vi "PXI-Update AO (Queue).vi"(0 "AO Tasks":T2[](array[typedef]), 5 "Wait for Buffer Space (T)?":bool=TRUE, 7 "AO Waveforms":dbl[][](array[numeric]), 11 "error in (no error)":errorcluster, 12 "DAQ Write State":T1) -> (14 "DAQ Write State Out":T1, 15 "error out":errorcluster)   [LabVIEW 2020]
uses:
  Type Defs/Task Struct.ctl
  Type Defs/DAQ Write State enum.ctl
  PXI Globals.vi
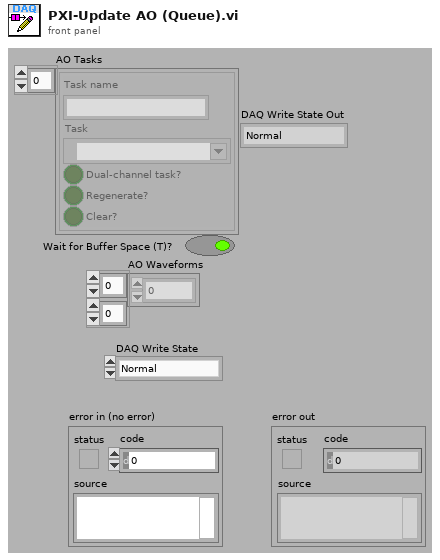
[diagram p1: front panel]
types:
  T1 = typedef "DAQ Write State enum.ctl" = enum16{"Normal", "Ramp down", "Zero buffers", "Done"}
  T2 = typedef "Task Struct.ctl" = cluster{"Task name":string, "Task":refnum<k21>, "Dual-channel task?":bool, "Regenerate?":bool, "Clear?":bool}
  T3 = typedef "Ramping Params.ctl" = cluster{"Ramp up?":bool, "Ramp down?":bool, "Ramp duration (msecs)":dbl, "Ramp type":enum16{"Linear", "Cos2"}}
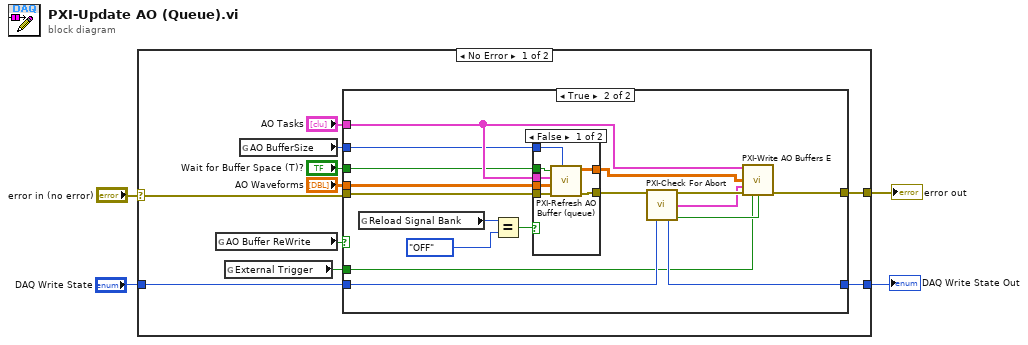
[diagram p0: block diagram]
diagram:
  n1 = case shown="No Error" "error in (no error)" {
    selector: "error in (no error)" -> [w11 w44]
    tunnel: [w14 w44] -> w4
    tunnel: "DAQ Write State" -> [w7 w43]
    tunnel: [w6 w43] -> w1
    frame No Error {
      n2 = global read "PXI Globals.vi" "AO Buffer ReWrite"() -> (w9:bool)
      n3 = global read "PXI Globals.vi" "External Trigger"() -> (w5:bool)
      n4 = global read "PXI Globals.vi" "AO BufferSize"() -> (w10:i32)
      n5 = case shown="True" w9 {
        tunnel: "AO Tasks" -> [_ w31]
        tunnel: w11 -> [w16 w30]
        tunnel: [w16 w32] -> w14
        tunnel: "AO Waveforms" -> [_ w33]
        tunnel: w10 -> [_ w27]
        tunnel: "Wait for Buffer Space (T)?" -> [_ w25]
        tunnel: w7 -> [w15 w22]
        tunnel: [w15 w19] -> w6
        tunnel: w5 -> [_ w17]
        frame False {
        }
        frame True {
          n6 = global read "PXI Globals.vi" "Reload Signal Bank"() -> (w28:enum32{"OFF", "ENABLED", "FORCED"})
          n7 = Equal?(x=w28, y=enum16{"OFF", "ENABLED", "FORCED"}."OFF") -> (x = y?=w26:bool)
          n8 = case shown="False" w26 {
            tunnel: w30 -> [w40 w42]
            tunnel: w33 -> [w39 w41]
            tunnel: [w38 w41] -> w18
            tunnel: [w37 w42] -> w24
            tunnel: w31 -> [w36 _]
            tunnel: w27 -> [w35 _]
            tunnel: w25 -> [w34 _]
            frame False {
              n9 = call "PXI-Refresh AO Buffer (queue).vi"("BufferSize"=w35, "error in (no error)"=w40, "AO Waveforms In"=w39, "AO Tasks"=w36, "Wait for buffer space? (T)"=w34) -> ("error out (no error)"=w37:errorcluster, "AO Waveforms Out"=w38:dbl[][])  [unwired: 5 in]
            }
            frame True {
            }
          }
          n10 = call "PXI-Check For Abort.vi"("error in (no error)"=w24, "DAQ Write State"=w22) -> ("error out"=w23:errorcluster, "Ramping"=w21:T3, "DAQ Write State Out"=w19:T1, "Zero?"=w20:bool)  [unwired: 10 in]
          n11 = call "PXI-Write AO Buffers E.vi"("AO Tasks"=w31, "AO Waveforms"=w18, "Ramping"=w21, "error in (no error)"=w23, "Force write"=w17, "zero output"=w20) -> ("error out"=w32:errorcluster)  [unwired: 8 in, 1 out]
        }
      }
    }
    frame Error {
    }
  }
  "error out" <- w4
  "DAQ Write State Out" <- w1
